vi "AOL Z Cal-Fine tuning sequence.vi"(9 "Max offset (us)":i32=10 min=5 max=100, 10 "Initial value":sgl=270.0 format="%#_13g") -> (1 "Ascending sequence":sgl[](array[numeric]), 3 "Descending sequence":sgl[](array[numeric]))   [LabVIEW 2017]
panel:
  in  "Negative first (F)":bool
  out "Offsets sequence":dbl[](array[numeric])
  out "size(s)":i32
  out "Calibration's optimised norm Z sequence":dbl[](array[numeric])
  out "Increment":dbl format="%#_12f"
  # "Recommended numbers of calibration points are 11, 21, 41 etc such as the increment step is always a nice value rounded to two decimal points."
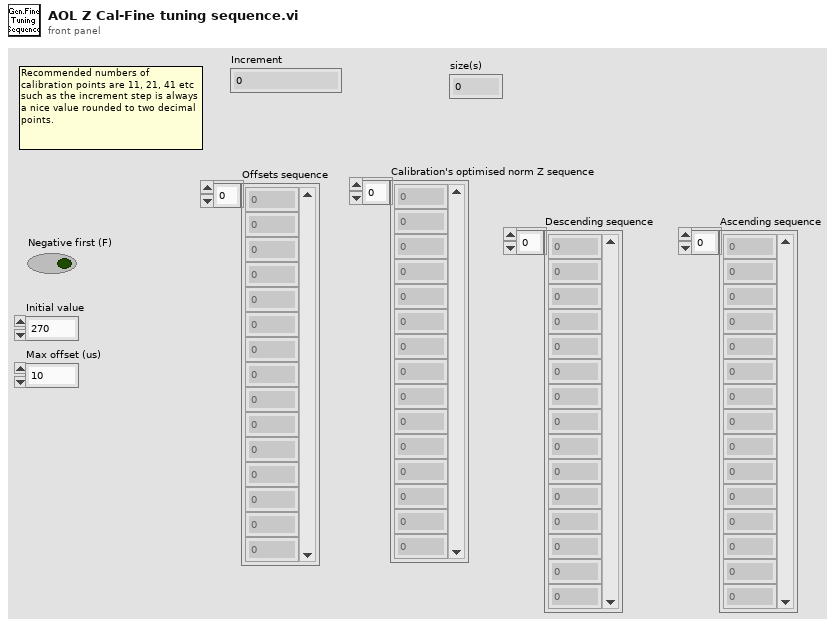
[diagram p1: front panel]
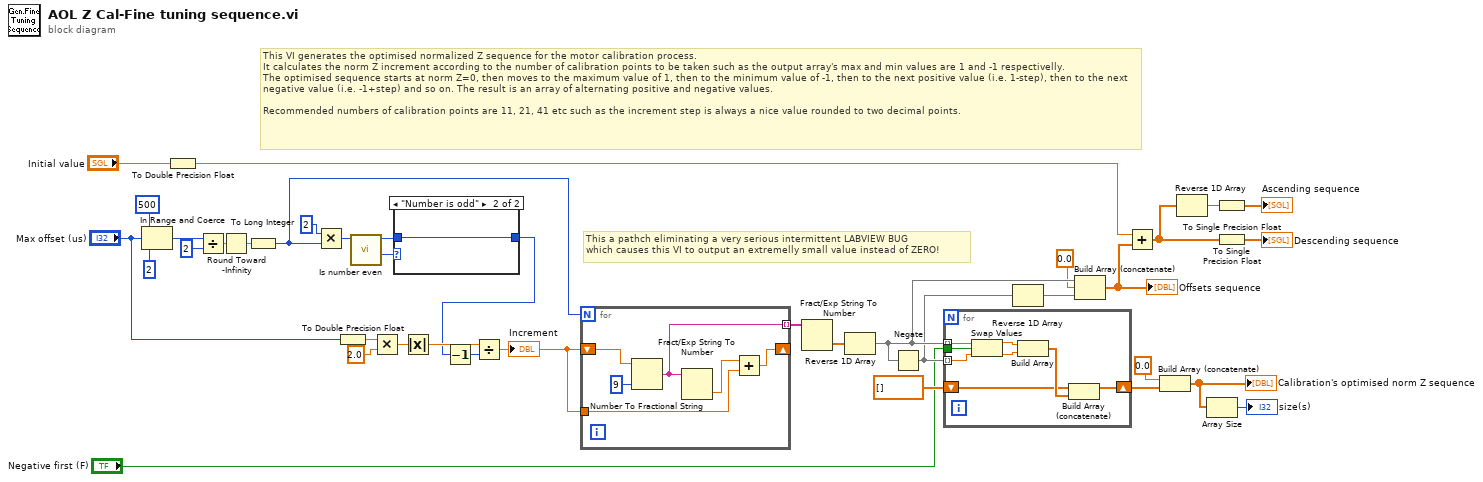
[diagram p0: block diagram]
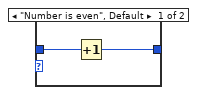
[diagram p2: hidden frame]
diagram:
  # "This VI generates the optimised normalized Z sequence for the motor calibration process.\nIt calculates the norm Z increment according to the number of calibration points to be taken such as the output array's max and min values are 1 and -1 respectivelly.\nThe optimised sequence starts at norm Z=0, then moves to the maximum value of 1, then to the minimum value of -1, then to the next positive value (i.e. 1-step), then to the next negative value (i.e. -1+step) and so on. The result is an array of alternating positive and negative values.\n\nRecommended numbers of calibration points are 11, 21, 41 etc such as the increment step is always a nice value rounded to two decimal points."
  # "This a pathch eliminating a very serious intermittent LABVIEW BUG\nwhich causes this VI to output an extremelly small value instead of ZERO!"
  n1 = In Range and Coerce(upper limit=500, x="Max offset (us)", lower limit=2) -> (coerced(x)=w19:i32)  [unwired: 1 out]
  n2 = To Double Precision Float(number="Initial value") -> (double precision float=w1:dbl)
  n3 = Divide(x=w19, y=2) -> (x/y=w32:dbl)
  n4 = Round Toward -Infinity(1:w32) -> (0:w25:dbl)
  n5 = To Long Integer(number=w25) -> (32bit integer=w17:i32)
  n6 = Multiply(x=2, y=w17) -> (x*y=w16:i32)
  n7 = To Double Precision Float(number="Max offset (us)") -> (double precision float=w4:dbl)
  n8 = call "Is number even.vi"("Number"=w16) -> ("Even/Odd"=w38:enum16{"Number is even", "Number is odd"}, "Number (dup)"=w15:i32)  [unwired: 9 in]
  n9 = Multiply(x=w4, y=2.0) -> (x*y=w30:dbl)
  n10 = case shown="\"Number is odd\"" w38 {
    tunnel: [w39 w41] -> w18
    tunnel: w15 -> [w40 w41]
    frame "Number is even", Default {
      n11 = Increment(x=w40) -> (x+1=w39:i32)
    }
    frame "Number is odd" {
    }
  }
  n12 = Absolute Value(x=w30) -> (abs(x)=w37:dbl)
  n13 = Decrement(x=w18) -> (x-1=w36:i32)
  n14 = Divide(x=w37, y=w36) -> (x/y=w34:dbl)
  "Increment" <- w34
  n15 = for {
    N: w17 -> [_]
    shift-right: [w46] -> _
    shift-left: w34 -> [w44]
    tunnel: w34 -> [w47]
    tunnel: [w42] -> w35 mode=indexing
    n16 = Number To Fractional String(number=w44, precision (6)=i16 9) -> (F-format string=w42:string)  [unwired: 2 in]
    n17 = Fract/Exp String To Number(string=w42) -> (number=w43:dbl)  [unwired: 3 in, 1 out]
    n18 = Add(x=w43, y=w47) -> (x+y=w46:dbl)
  }
  n19 = Fract/Exp String To Number(string=w35) -> (number=w28:dbl[])  [unwired: 3 in, 1 out]
  n20 = Reverse 1D Array(array=w28) -> (reversed array=w14:dbl[])
  n21 = Negate(x=w14) -> (-x=w13:dbl[])
  n22 = for {
    tunnel: w14 -> [w52] mode=indexing
    tunnel: w13 -> [w51] mode=indexing
    shift-right: [w54] -> w26
    shift-left: dbl[] [] -> [w53]
    tunnel: "Negative first (F)" -> [w48]
    n23 = Swap Values(12:w52, 13:w48, 14:w51) -> (1:w49:dbl, 3:w50:dbl)
    n24 = Build Array(w49, w50) -> (w55:dbl[])
    n25 = Build Array (concatenate)(w53, w55) -> (w54:dbl[])
  }
  n26 = Reverse 1D Array(array=w13) -> (reversed array=w12:dbl[])
  n27 = Build Array (concatenate)(w14, 0.0 ("x/y"), w12) -> (w9:dbl[])
  "Offsets sequence" <- w9
  n28 = Add(x=w1, y=w9) -> (x+y=w6:dbl[])
  n29 = Build Array (concatenate)(0.0 ("x/y"), w26) -> (w24:dbl[])
  "Calibration's optimised norm Z sequence" <- w24
  n30 = Reverse 1D Array(array=w6) -> (reversed array=w7:dbl[])
  n31 = Array Size(array=w24) -> (size(s)=→"size(s)":i32)
  n32 = To Single Precision Float(number=w7) -> (single precision float=→"Ascending sequence":sgl[])
  n33 = To Single Precision Float(number=w6) -> (single precision float=→"Descending sequence":sgl[])
